vi "Register Emitters.vi"(8 "error in":errorcluster, 10 "Emitter":string, 11 "Controller in":refnum<class "Controller.lvclass">) -> (0 "error out":errorcluster, 3 "Controller out":refnum<class "Controller.lvclass">)   [LabVIEW 2014, in "Controller.lvlib" / "Controller.lvclass"]
uses:
  Controller.lvclass
  Controller.lvclass/Controller.ctl
  reusable/Data/Data.lvclass
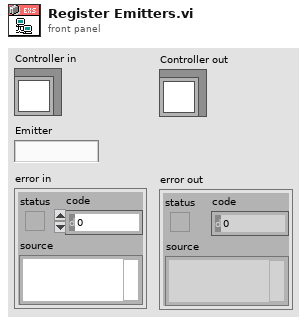
[diagram p1: front panel]
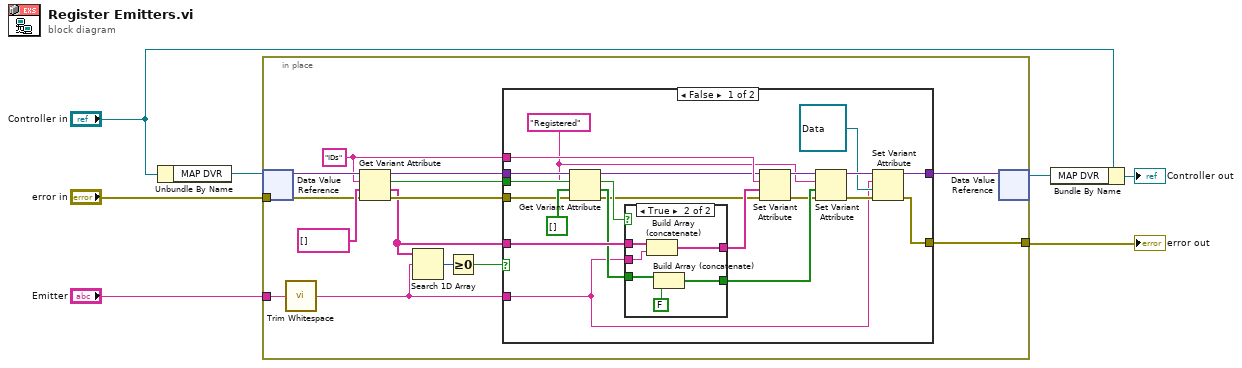
[diagram p0: block diagram]
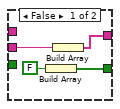
[diagram p2: hidden frame]
diagram:
  n1 = Unbundle By Name("Controller in") -> ("MAP DVR"=w7:refnum<data-value>)
  n2 = in-place {
    in-place-border: "Emitter" -> [w12]
    in-place-border: "error in" -> [w15]
    in-place-border: [w13] -> w1
    w18 = "IDs" ("name")
    n3 = in-place-dvr #1(w7) -> (w21:variant)  [unwired: 1 out]
    n4 = call <vilib>:"Trim Whitespace.vi"("string"=w12) -> ("trimmed string"=w10:string)  [unwired: 1 in]
    n5 = Get Variant Attribute(Variant=w21, name=w18, default value (empty Variant)=string[] [], error in=w15) -> (duplicate Variant=w17:variant, found=w19:bool, value=w11:string[], error out=w16:errorcluster)
    n6 = Search 1D Array(1D array=w11, element=w10) -> (index of element=w9:i32)  [unwired: 1 in]
    n7 = Greater Or Equal To 0?(x=w9) -> (x >= 0?=w8:bool)
    n8 = case shown="False" w8 {
      tunnel: w19 -> [w41 _]
      tunnel: w11 -> [w40 _]
      tunnel: w18 -> [w39 _]
      tunnel: w17 -> [w36 w53]
      tunnel: w16 -> [w28 w52]
      tunnel: [w24 w53] -> w14
      tunnel: [w23 w52] -> w13
      tunnel: w10 -> [w22 _]
      frame False {
        w31 = "Registered" ("name")
        n9 = Get Variant Attribute(Variant=w36, name=w31, default value (empty Variant)=bool[] [], error in=w28) -> (duplicate Variant=w35:variant, value=w34:bool[], error out=w29:errorcluster)  [unwired: 1 out]
        n10 = case shown="True" w41 {
          tunnel: w40 -> [_ w51]
          tunnel: w22 -> [w45 w50]
          tunnel: [w44 w49] -> w38
          tunnel: w34 -> [_ w48]
          tunnel: [w42 w47] -> w33
          frame False {
            n11 = Build Array(FALSE) -> (w42:bool[])
            n12 = Build Array(w45) -> (w44:string[])
          }
          frame True {
            n13 = Build Array (concatenate)(w51, w50) -> (w49:string[])
            n14 = Build Array (concatenate)(w48, FALSE) -> (w47:bool[])
          }
        }
        n15 = Set Variant Attribute(Variant=w35, name=w39, value=w38, error in=w29) -> (Variant out=w32:variant, error out=w30:errorcluster)  [unwired: 1 out]
        n16 = Set Variant Attribute(Variant=w32, name=w31, value=w33, error in=w30) -> (Variant out=w27:variant, error out=w26:errorcluster)  [unwired: 1 out]
        n17 = Set Variant Attribute(Variant=w27, name=w22, value=refnum<class "Data.lvclass"> refnum ("Base Data Lib:Data"), error in=w26) -> (Variant out=w24:variant, error out=w23:errorcluster)  [unwired: 1 out]
      }
      frame True {
        # "Emitters can already be registered if an actor is launched and returning data before this is run.  Prevent multiple registration..."
      }
    }
    n18 = in-place-dvr #1(w14) -> (w4:refnum<data-value>)  [unwired: 1 out]
  }
  "error out" <- w1
  n19 = Bundle By Name(cluster="Controller in", "MAP DVR"=w4) -> (→"Controller out":refnum<class "Controller.lvclass">)
